vi "CountingBoard.vi"() -> ()   [LabVIEW 2018]
uses:
  <vilib>/MakerHub/LINX/Public/Peripherals/Digital/Digital Write N Chans.vi
  <vilib>/MakerHub/LINX/Private/Local IO/LinxDigitalWrite.vi
  <vilib>/MakerHub/LINX/Public/Utilities/Check Channel.vi
  <vilib>/MakerHub/LINX/Public/Utilities/Open Serial.vi
  <vilib>/MakerHub/LINX/Private/Utilties/Generate Error.vi
  <vilib>/MakerHub/LINX/LMH-LINX.lvlib
panel:
  out "Arduino State":bool[](array[boolean])
  in  "D0 Channels":u8[](array[numeric])=[2, 3, 4, 5]
  in  "Stop Button":bool
  in  "Serial Port":refnum<visa-resource-name>
  out "Squared Number (Py)":dbl
  in  "Python Path":path
  out "Counted to":dbl
  out "Finished":bool
  out "Counting":bool
  out "Squared Number (LV)":dbl
  in  "Input":dbl
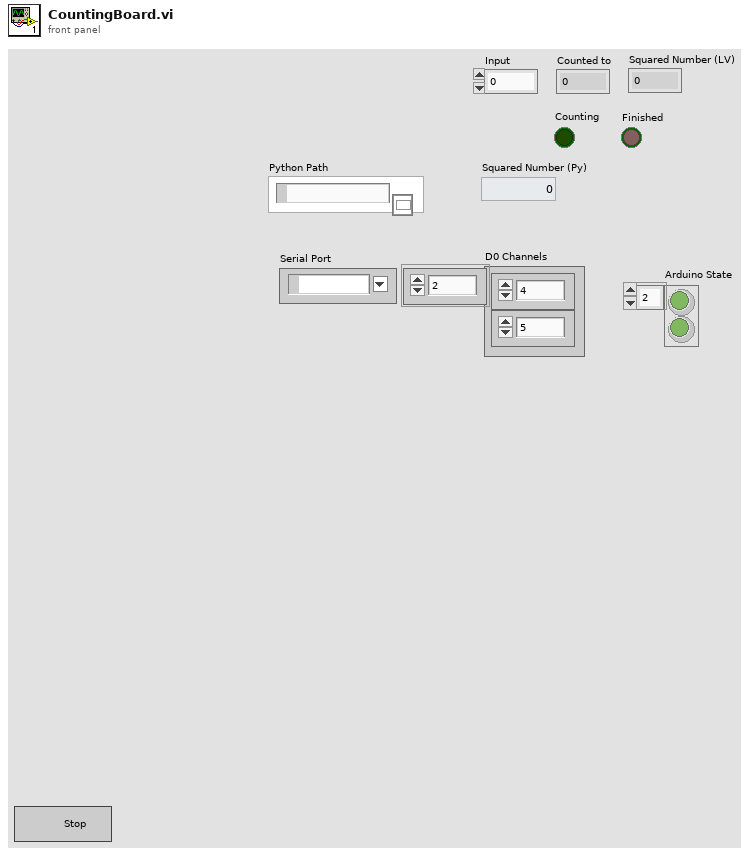
[diagram p1: front panel]
types:
  T1 = typedef "LMH-LINX.lvlib/LINX Ref.ctl" = cluster{"IO":T2, "Interface":T3, "LINX Device Config":T4}
  T2 = typedef "LMH-LINX.lvlib/Platform.ctl" = enum16{"Remote", "Local"}
  T3 = typedef "LMH-LINX.lvlib/Interface.ctl" = enum16{"Serial", "TCP"}
  T4 = typedef "LMH-LINX.lvlib/Device.lvlib/LINX Device Config.ctl" = cluster{"Interface":T3, "COM Port":refnum<visa-resource-name>, "TCP Configuration":T5, "Device Family":u8, "Device ID":u8, "Device Name":string, "TCP Ref":refnum<k5>, "Channels":T6}
  T5 = typedef "LMH-LINX.lvlib/Device.lvlib/TCP Config.ctl" = cluster{"IP Address":string, "Port":u16}
  T6 = typedef "LMH-LINX.lvlib/Channels.ctl" = cluster{"DI":u8[], "DO":u8[], "AI":u8[], "AO":u8[], "PWM":u8[], "QE":u8[], "UART":u8[], "I2C 2":u8[], "SPI":u8[], "CAN":u8[], "Servo":u8[], "AI Ref (V)":dbl, "AI Resolution (Bits)":u8, "AO Ref (V)":dbl, "AO Resolution (Bits)":u8}
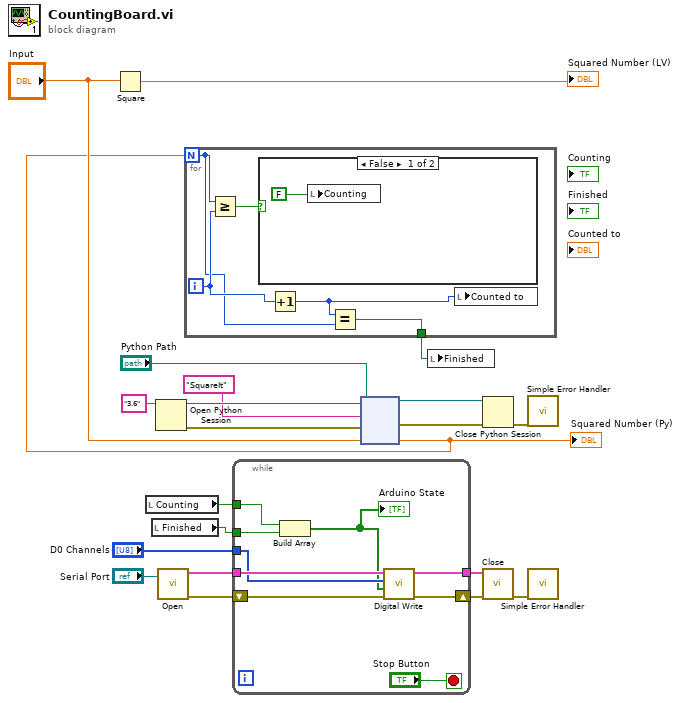
[diagram p0: block diagram]
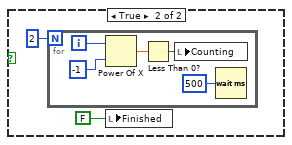
[diagram p2: hidden frame]
diagram:
  n1 = Square(x="Input") -> (x^2=→"Squared Number (LV)":dbl)
  n2 = local read "Counting"() -> (w5:bool)
  n3 = local read "Finished"() -> (w4:bool)
  n4 = Open Python Session(python version="3.6" ("Python version")) -> (session out=w19:refnum<k35>, error out=w21:errorcluster)  [unwired: 2 in]
  n5 = call-poly <vilib>:"Open.vi"("Serial Port"="Serial Port") -> ("Error Out"=w11:errorcluster, "LINX Resource"=w12:T1)  [unwired: 8 in, 1 out]
  n6 = while {
    tunnel: w12 -> [w28]
    tunnel: [w29] -> w10
    shift-right: [w30] -> w9
    shift-left: w11 -> [w27]
    tunnel: "D0 Channels" -> [w25]
    tunnel: w5 -> [w24]
    tunnel: w4 -> [w23]
    stop <- "Stop Button" stop-if-true
    n7 = Build Array(w24, w23) -> (w22:bool[])
    "Arduino State" <- w22
    n8 = call-poly <vilib>:"Digital Write.vi"("Error In"=w27, "Values"=w22, "DO Channels"=w25, "LINX Resource"=w28) -> ("Error Out"=w30:errorcluster, "LINX Resource"=w29:T1)  [unwired: 6 in]
  }
  n9 = node(w19, "Python Path", "SquareIt" ("function name"), w21, "Input") -> (w18:refnum<k35>, w20:errorcluster, w1:dbl)  [unwired: 2 in, 2 out]
  "Squared Number (Py)" <- w1
  n10 = for {
    N: w1 -> [w32]
    tunnel: [w31] -> w2
    i -> [w34]
    n11 = Greater Or Equal?(x=w32, y=w34) -> (x >= y?=w35:bool)
    n12 = case shown="False" w35 {
      frame False {
        n13 = local write "Counting"(FALSE) -> ()
      }
      frame True {
        n14 = for {
          N: 2 -> [_]
          i -> [w40]
          n15 = Power Of X(1:-1, 2:w40) -> (0:w42:dbl)
          n16 = Less Than 0?(x=w42) -> (x < 0?=w41:bool)
          n17 = local write "Counting"(w41) -> ()
          n18 = Wait (ms)(milliseconds to wait=u32 500) -> ()  [unwired: 1 out]
        }
        n19 = local write "Finished"(FALSE) -> ()
      }
    }
    n20 = Increment(x=w34) -> (x+1=w33:i32)
    n21 = Equal?(x=w33, y=w32) -> (x = y?=w31:bool)
    n22 = local write "Counted to"(w33) -> ()
  }
  n23 = local write "Finished"(w2) -> ()
  n24 = Close Python Session(session in=w18, error in=w20) -> (11:w14:errorcluster)
  n25 = call <vilib>:"Close.vi"("Error In"=w9, "LINX Resource"=w10) -> ("Error Out"=w7:errorcluster)  [unwired: 9 in]
  n26 = call <vilib>:"Simple Error Handler.vi"("error in (no error)"=w14) -> ()  [unwired: 4 in, 5 out]
  n27 = call <vilib>:"Simple Error Handler.vi"("error in (no error)"=w7) -> ()  [unwired: 4 in, 5 out]
